vi "Modbus.vi"() -> ()   [LabVIEW 2017]
uses:
  <vilib>/NI Modbus.llb/MB Ethernet Master Query Write Multiple Registers (poly).vi
  <vilib>/NI Modbus.llb/MB Ethernet Master Query Write Multiple Coils (poly).vi
panel:
  in  "Coils":bool[](array[boolean])
  out "error out":errorcluster
  in  "Starting Address":u16
  in  "Registers":u16[](array[numeric])
  in  "remote port or service name":u16
  in  "address":string
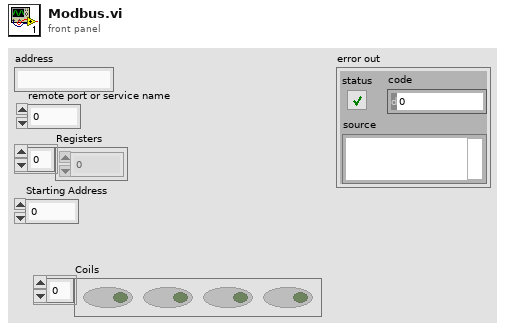
[diagram p1: front panel]
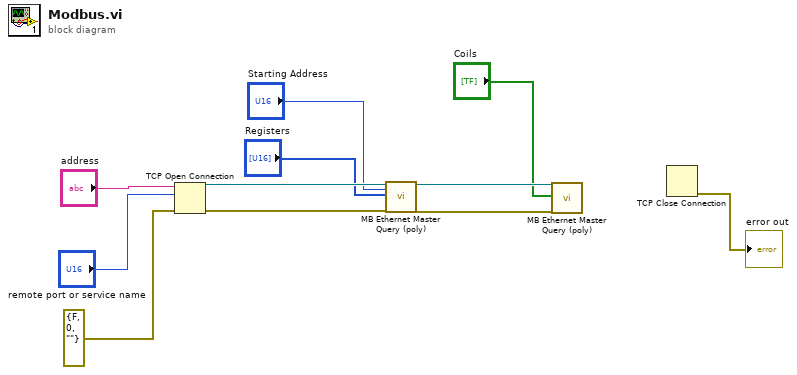
[diagram p0: block diagram]
diagram:
  n1 = TCP Open Connection(address="address", remote port or service name="remote port or service name", error in (no error)=errorcluster {"status"=FALSE, "code"=0, "source"=""}) -> (connection ID=w7:refnum<k5>, error out=w8:errorcluster)  [unwired: 2 in]
  n2 = call-poly <vilib>:"MB Ethernet Master Query (poly).vi"("TCP Connection Refnum in"=w7, "Starting Address"="Starting Address", "Registers"="Registers", "error in"=w8) -> ("TCP Connection Refnum (dup)"=w2:refnum<k5>, "error out"=w3:errorcluster)  [unwired: 13 in, 1 out]
  n3 = call-poly <vilib>:"MB Ethernet Master Query (poly).vi"("TCP Connection Refnum in"=w2, "Coils"="Coils", "error in"=w3) -> ()  [unwired: 14 in, 3 out]
  n4 = TCP Close Connection() -> (error out=→"error out":errorcluster)  [unwired: 3 in, 1 out]
